vi "Initialize Custom Events.vi"   [LabVIEW 2013]
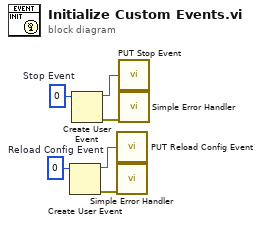
[diagram p0: block diagram]
diagram:
  w1 = 0  # Reload Config Event
  w6 = 0  # Stop Event
  n1 = Create User Event(user event datatype=w1) -> (user event=w2:refnum<user-event>, error out=w3:errorcluster)  [unwired: 1 in]
  n2 = Create User Event(user event datatype=w6) -> (user event=w5:refnum<user-event>, error out=w4:errorcluster)  [unwired: 1 in]
  n3 = call "PUT Reload Config Event.vi"("Reload Config Event"=w2) -> ()
  n4 = call <vilib>:"Simple Error Handler.vi"("error in (no error)"=w3) -> ()  [unwired: 4 in, 5 out]
  n5 = call "PUT Stop Event.vi"("Stop Event"=w5) -> ()
  n6 = call <vilib>:"Simple Error Handler.vi"("error in (no error)"=w4) -> ()  [unwired: 4 in, 5 out]
